vi "Get Virtual Devices.vi"(8 "error in":errorcluster) -> (0 "error out":errorcluster, 3 "Virtual Devices":string[](array[string]))   [LabVIEW 2023, in "SwitchExecController.lvlib"]
uses:
  SwitchExecController.lvlib
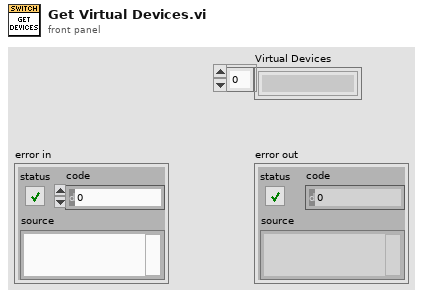
[diagram p1: front panel]
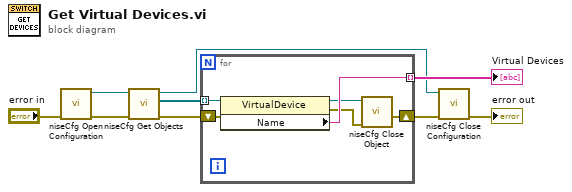
[diagram p0: block diagram]
diagram:
  n1 = call <vilib>:"niseCfg Open Configuration.vi"("error in (no error)"="error in") -> ("error out"=w8:errorcluster, "niseCfg"=w7:refnum<k7>)  [unwired: 9 in]
  n2 = call-poly <vilib>:"niseCfg Get Objects.vi"("error in (no error)"=w8, "niseCfg"=w7) -> ("error out"=w1:errorcluster, "Virtual Devices"=w4:refnum<k7>[], "niseCfg out"=w2:refnum<k7>)  [unwired: 7 in]
  n3 = for {
    tunnel: w4 -> [w15] mode=indexing
    tunnel: [w14] -> w9 mode=indexing
    shift-right: [w10] -> w5
    shift-left: w1 -> [w13]
    n4 = property class="VirtualDevice"(reference=w15, error in=w13) -> (reference out=w12:refnum<k7>, error out=w11:errorcluster, "Name"=w14:string)
    n5 = call <vilib>:"niseCfg Close Object.vi"("error in (no error)"=w11, "Reference"=w12) -> ("error out"=w10:errorcluster)  [unwired: 9 in]
  }
  "Virtual Devices" <- w9
  n6 = call <vilib>:"niseCfg Close Configuration.vi"("error in (no error)"=w5, "niseCfg"=w2) -> ("error out"=→"error out":errorcluster)  [unwired: 9 in]
